vi "Dialog Properties.vi"(8 "Error In (No Error)":errorcluster, 10 "Enable Dialog Properties":bool, 11 "VI Ref  In":refnum<vi>) -> (0 "Error Out":errorcluster, 3 "VI Ref Out":refnum<vi>)   [LabVIEW 2024]
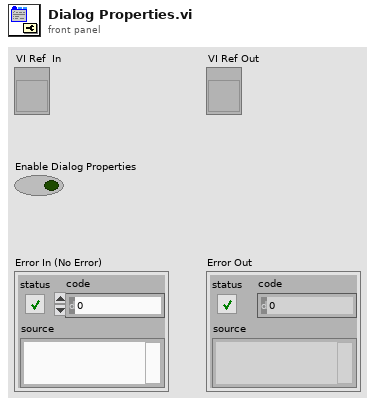
[diagram p1: front panel]
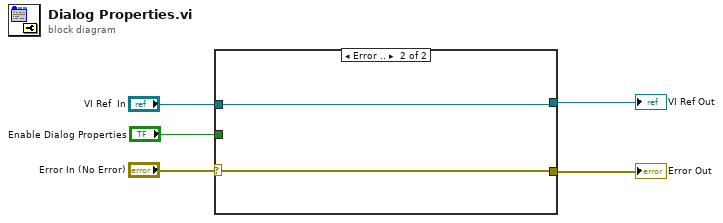
[diagram p0: block diagram]
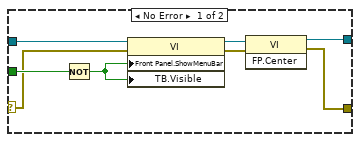
[diagram p2: hidden frame]
diagram:
  n1 = case shown="Error .." "Error In (No Error)" {
    selector: "Error In (No Error)" -> [w6 w14]
    tunnel: [w13 w14] -> w5
    tunnel: "VI Ref  In" -> [w12 w15]
    tunnel: "Enable Dialog Properties" -> [w8 _]
    tunnel: [w9 w15] -> w2
    frame No Error {
      n2 = Not(x=w8) -> (.not. x?=w7:bool)
      n3 = property class="VI"(reference=w12, error in=w6, "Front Panel.ShowMenuBar"=w7, "TB.Visible"=w7) -> (reference out=w10:refnum<vi>, error out=w11:errorcluster)
      n4 = invoke class="VI" method="FP.Center"(reference=w10, error in=w11) -> (reference out=w9:refnum<vi>, error out=w13:errorcluster)  [unwired: 1 in, 1 out]
    }
    frame Error {
    }
  }
  "Error Out" <- w5
  "VI Ref Out" <- w2
